vi "GetVoltage.vi"(4 "error in":errorcluster, 5 "connection ID":refnum<k5>) -> (0 "Voltage":string, 1 "error out":errorcluster, 2 "connection ID out":refnum<k5>, 3 "Answer":bool)   [LabVIEW 2013]
panel:
  out "читаю hex":string
  out "читаю текст":string
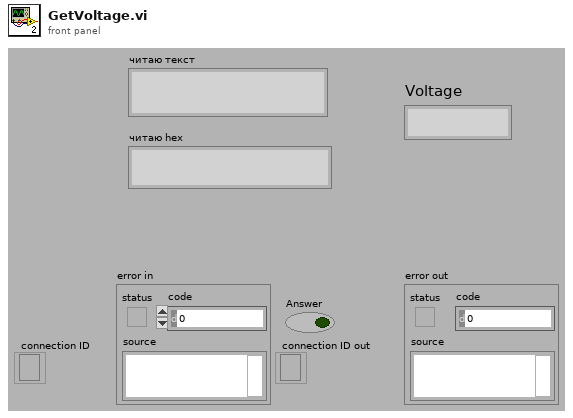
[diagram p1: front panel]
types:
  T1 = enum16{"Standard", "Buffered", "CRLF", "Immediate"}
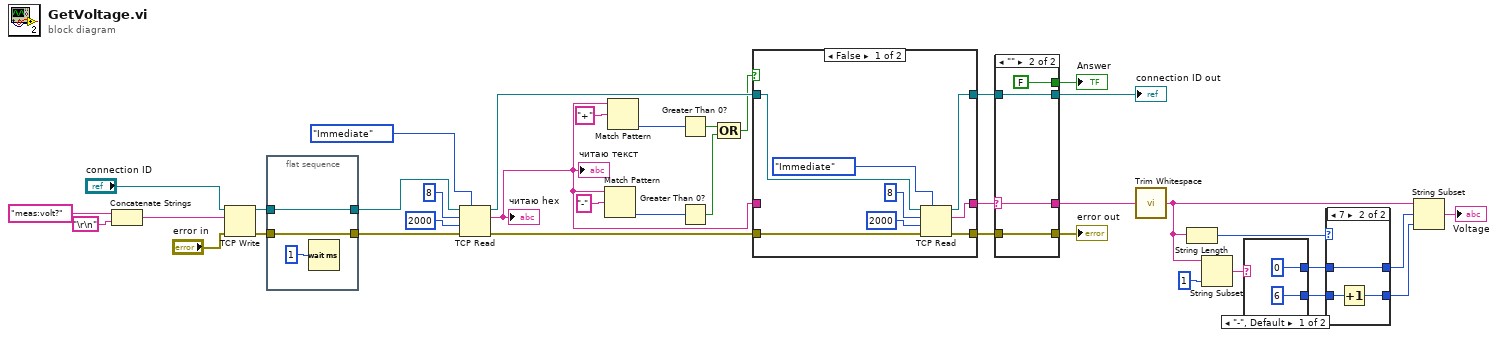
[diagram p0: block diagram]
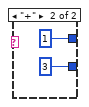
[diagram p3: hidden frame]
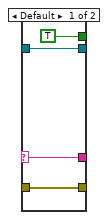
[diagram p5: hidden frame]
diagram:
  n1 = Concatenate Strings("meas:volt?" ("data in"), "\r\n") -> (w35:string)
  n2 = TCP Write(connection ID="connection ID", data in=w35, error in (no error)="error in") -> (connection ID out=w28:refnum<k5>, error out=w30:errorcluster)  [unwired: 2 out]
  n3 = flat-sequence {
    tunnel: [w41] -> w29
    tunnel: w30 -> [w41]
    tunnel: [w40] -> w27
    tunnel: w28 -> [w40]
    frame #0 {
      n4 = Wait (ms)(milliseconds to wait=u32 1) -> ()  [unwired: 1 out]
    }
  }
  n5 = TCP Read(connection ID=w27, bytes to read=8, error in (no error)=w29, 7:T1."Immediate" ("mode (standard)"), 9:2000 ("timeout ms (25000)")) -> (connection ID out=w18:refnum<k5>, data out=w15:string, error out=w19:errorcluster)
  "читаю hex" <- w15
  "читаю текст" <- w15
  n6 = Match Pattern(string=w15, regular expression="-") -> (offset past match=w14:i32)  [unwired: 1 in, 3 out]
  n7 = Match Pattern(string=w15, regular expression="+") -> (offset past match=w25:i32)  [unwired: 1 in, 3 out]
  n8 = Greater Than 0?(x=w25) -> (x > 0?=w13:bool)
  n9 = Greater Than 0?(x=w14) -> (x > 0?=w12:bool)
  n10 = Compound Arithmetic op=OR(w13, w12) -> (w11:bool)
  n11 = case shown="False" w11 {
    tunnel: w15 -> [_ w52]
    tunnel: [w46 w52] -> w21
    tunnel: [w44 w50] -> w20
    tunnel: w19 -> [w45 w50]
    tunnel: w18 -> [w47 w51]
    tunnel: [w42 w51] -> w17
    frame False {
      n12 = TCP Read(connection ID=w47, bytes to read=8, error in (no error)=w45, 7:T1."Immediate" ("mode (standard)"), 9:2000 ("timeout ms (25000)")) -> (connection ID out=w42:refnum<k5>, data out=w46:string, error out=w44:errorcluster)
    }
    frame True {
    }
  }
  n13 = case shown="\"\"" w21 {
    selector: w21 -> [w56 w60]
    tunnel: [w56 w60] -> w1
    tunnel: [TRUE FALSE] -> w22
    tunnel: w20 -> [w54 w58]
    tunnel: [w54 w58] -> w23
    tunnel: w17 -> [w53 w57]
    tunnel: [w53 w57] -> w24
    frame Default {
    }
    frame "" {
    }
  }
  "Answer" <- w22
  "connection ID out" <- w24
  "error out" <- w23
  n14 = call <vilib>:"Trim Whitespace.vi"("string"=w1) -> ("trimmed string"=w8:string)  [unwired: 1 in]
  n15 = String Length(string=w8) -> (length=w7:i32)
  n16 = String Subset(string=w8, length (rest)=1 ("length (rest)")) -> (substring=w10:string)  [unwired: 1 in]
  n17 = case shown="\"-\", Default" w10 {
    tunnel: [0 ("length (rest)") 1 ("length (rest)")] -> w4
    tunnel: [6 ("length (rest)") 3 ("length (rest)")] -> w6
    frame "-", Default {
    }
    frame "+" {
    }
  }
  n18 = case shown="7" w7 {
    tunnel: w6 -> [w66 w69]
    tunnel: [w66 w68] -> w5
    tunnel: w4 -> [w65 w67]
    tunnel: [w65 w67] -> w3
    frame 6, Default {
    }
    frame 7 {
      n19 = Increment(x=w69) -> (x+1=w68:i32)
    }
  }
  n20 = String Subset(string=w8, offset (0)=w3, length (rest)=w5) -> (substring=→"Voltage":string)
